vi "Drive Motor Control Test.vi"() -> ()   [LabVIEW 2009]
uses:
  Motor Output Global.vi
  Motor Encoder Global.vi
  Inner Control/Drive Control Global DO NOT MODIFY!.vi
panel:
  in  "Manual Override?":bool
  in  "stop":bool
  in  "Drive Speed Control Feedback Gain":fxp<+/-,13,4>
  in  "Drive Speed Set Point (ft/sec)":fxp<+/-,18,8>
  in  "Drive Enable":bool
  out "Drive Encoder ft/sec":fxp<+/-,18,8>
  out "Drive Encoder tick/count":u32
  out "Drive Encoder":i32
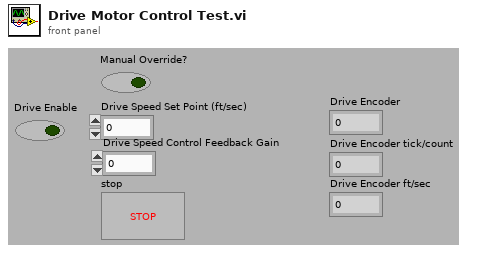
[diagram p1: front panel]
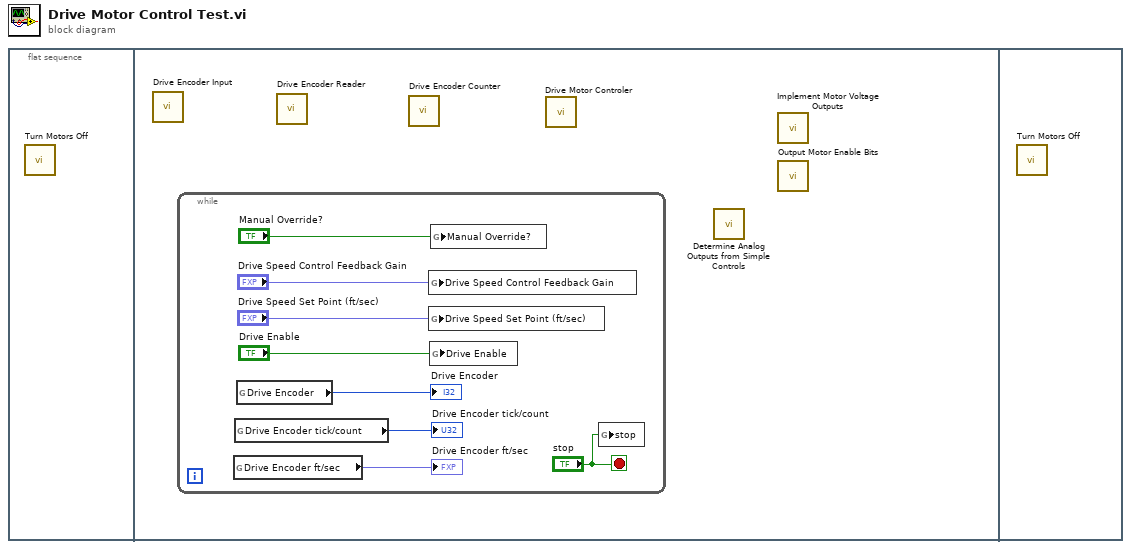
[diagram p0: block diagram]
diagram:
  n1 = flat-sequence {
    frame #0 {
      n2 = call "Turn Motors Off.vi"() -> ()  [unwired: 1 in]
    }
    frame #1 {
      n3 = call "Drive Encoder Input.vi"() -> ()  [unwired: 1 in]
      n4 = while {
        stop <- "stop" stop-if-true
        n5 = global read "Drive Control Global DO NOT MODIFY!.vi" "Drive Encoder ft/sec"() -> (→"Drive Encoder ft/sec":fxp<+/-,18,8>)
        n6 = global read "Drive Control Global DO NOT MODIFY!.vi" "Drive Encoder tick/count"() -> (→"Drive Encoder tick/count":u32)
        n7 = global read "Motor Encoder Global.vi" "Drive Encoder"() -> (→"Drive Encoder":i32)
        n8 = global write "Motor Encoder Global.vi" "Drive Speed Control Feedback Gain"("Drive Speed Control Feedback Gain") -> ()
        n9 = global write "Motor Encoder Global.vi" "Drive Speed Set Point (ft/sec)"("Drive Speed Set Point (ft/sec)") -> ()
        n10 = global write "Motor Output Global.vi" "Drive Enable"("Drive Enable") -> ()
        n11 = global write "Motor Output Global.vi" "Manual Override?"("Manual Override?") -> ()
        n12 = global write "Motor Encoder Global.vi" "stop"("stop") -> ()
      }
      n13 = call "Drive Encoder Reader.vi"() -> ()  [unwired: 1 in]
      n14 = call "Drive Encoder Counter.vi"() -> ()  [unwired: 1 in]
      n15 = call "Drive Motor Controler.vi"() -> ()  [unwired: 1 in]
      n16 = call "Determine Analog Outputs from Simple Controls.vi"() -> ()  [unwired: 1 in]
      n17 = call "Implement Motor Voltage Outputs.vi"() -> ()  [unwired: 1 in]
      n18 = call "Output Motor Enable Bits.vi"() -> ()  [unwired: 1 in]
    }
    frame #2 {
      n19 = call "Turn Motors Off.vi"() -> ()  [unwired: 1 in]
    }
  }
